vi "Main.vi"() -> ()   [LabVIEW 2020]
uses:
  <vilib>/Instr/_visa.llb/VISA Configure Serial Port (Instr).vi
panel:
  out "Boolean 8":bool=TRUE
  out "Numeric 4":dbl
  out "Numeric 2":dbl
  out "Numeric":dbl
  out "Boolean 7":bool=TRUE
  out "Boolean 6":bool
  out "Boolean 5":bool
  out "Boolean 4":bool
  out "Boolean 3":bool
  out "Boolean 2":bool
  out "Boolean":bool=TRUE
  out "NewVal":bool
  in  "Transmit":bool
  out "Transmitted Data":T1 {"LED" format="%04b"}
  in  "Period":u32
  out "data string":string
  out "Motor Speed":T2(graph)
  out "Waveform Chart":T3(graph)
  out "read buffer":string
  out "Received Data":cluster{i32[], u32}
  in  "Data to transmit":T1 {"LED" format="%04b"}
  out "error out":errorcluster
  in  "VISA resource name":refnum<visa-resource-name>
  in  "Stop":bool
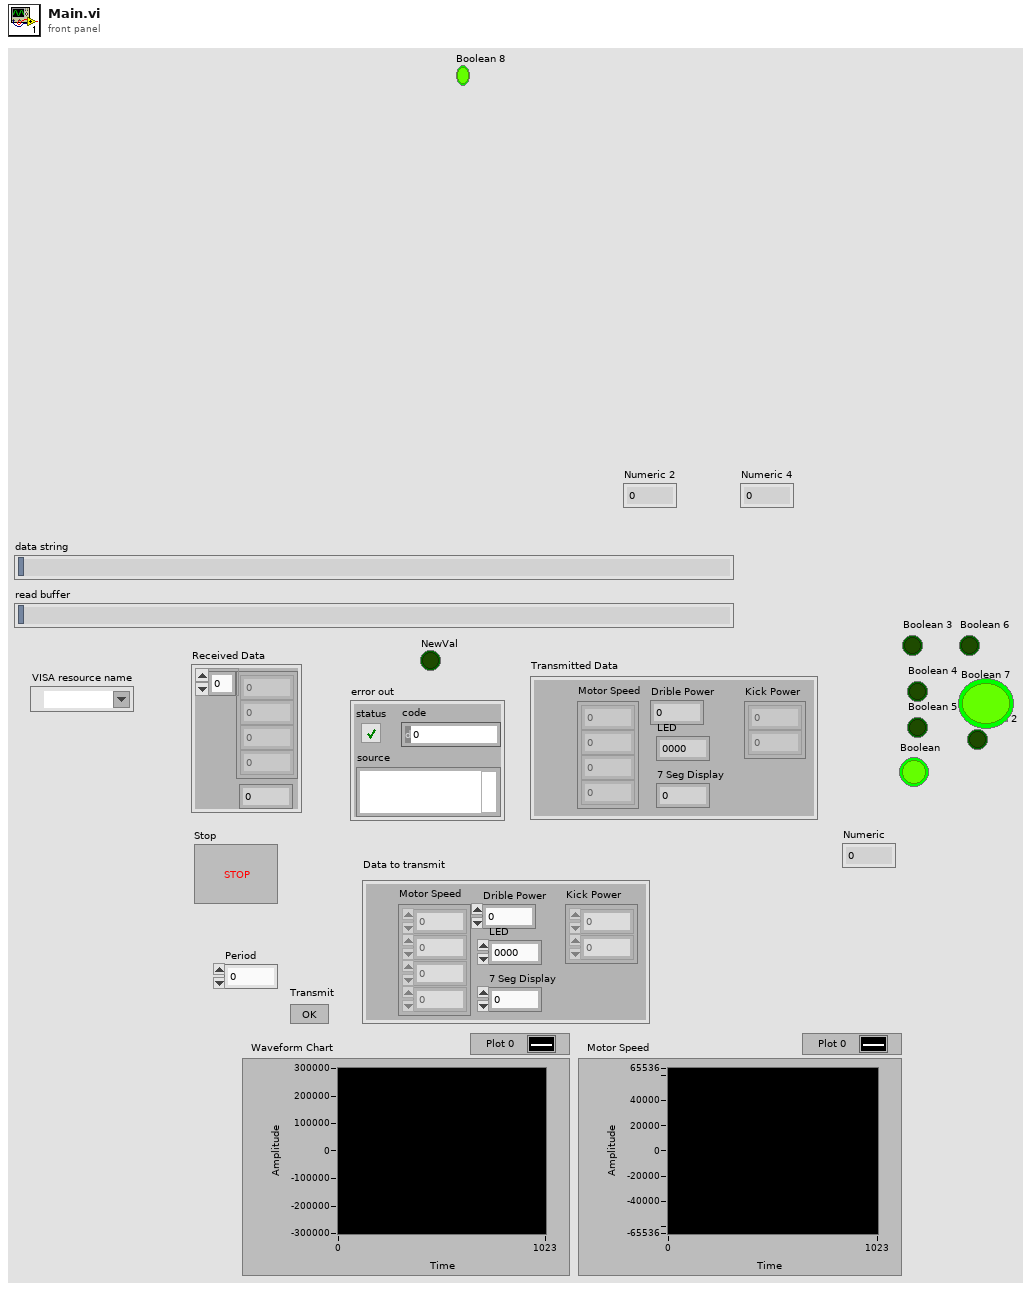
[diagram p1: front panel]
types:
  T1 = cluster{"Motor Speed":i32[], "Drible Power":i32, "LED":u32, "7 Seg Display":u32, "Kick Power":u32[]}
  T2 = cluster{"Motor Speed[0]":i32, "Motor Speed[1]":i32, "Motor Speed[2]":i32, "Motor Speed[3]":i32}
  T3 = cluster{"Encoder[0]":i32, "Encoder[1]":i32, "Encoder[2]":i32, "Encoder[3]":i32}
  T4 = enum16{"big-endian, network order", "native, host order", "little-endian"}
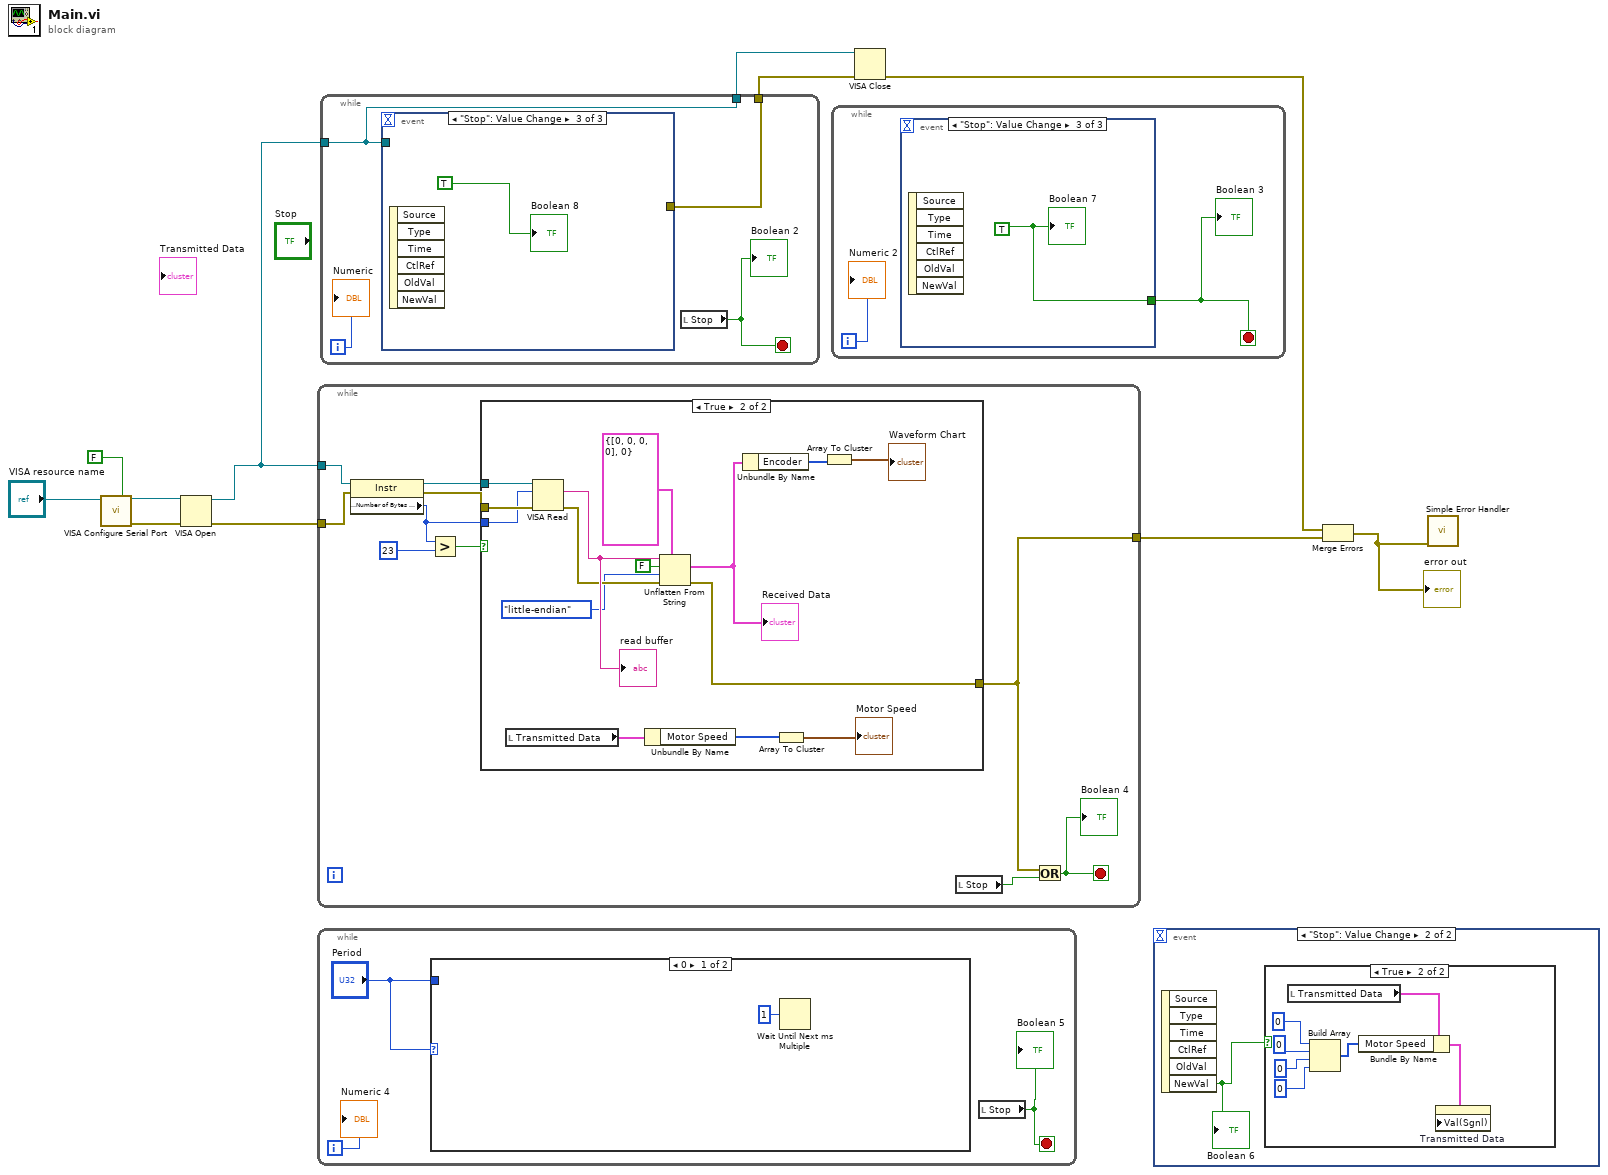
[diagram p0: block diagram]
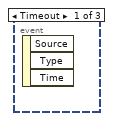
[diagram p2: hidden frame]
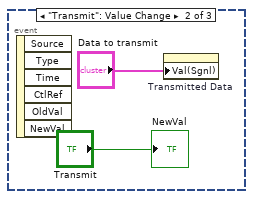
[diagram p3: hidden frame]
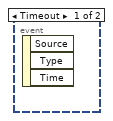
[diagram p4: hidden frame]
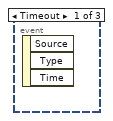
[diagram p6: hidden frame]
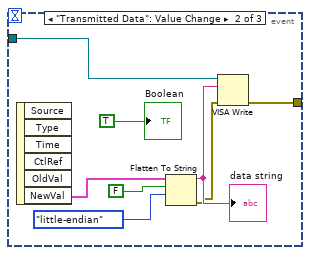
[diagram p7: hidden frame]
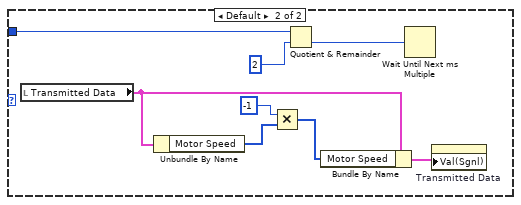
[diagram p9: hidden frame]
diagram:
  n1 = call-poly "VISA Configure Serial Port"("VISA resource name"="VISA resource name", "Enable Termination\nChar (T)"=FALSE ("Enable Termination\nChar (T)")) -> ("VISA resource name out"=w4:refnum<visa-resource-name>, "error out"=w2:errorcluster)  [unwired: 12 in]
  n2 = VISA Open(error in (no error)=w2, VISA resource name=w4) -> (VISA resource name=w10:refnum<visa-resource-name>, error out=w11:errorcluster)  [unwired: 3 in]
  n3 = while {
    tunnel: w10 -> [w17]
    tunnel: w11 -> [w16]
    tunnel: [w13] -> w6
    stop <- w12 stop-if-true
    n4 = property class="Instr"(reference=w17, error in=w16) -> (reference out=w19:refnum<visa-resource-name>, error out=w18:errorcluster, "Serial Settings:Number of Bytes at Serial Port"=w15:u32)
    n5 = Greater?(x=w15, y=u32 23) -> (0:w20:bool)
    n6 = case shown="True" w20 {
      tunnel: w19 -> [_ w37]
      tunnel: w18 -> [w22 w34]
      tunnel: [w22 w32] -> w13
      tunnel: w15 -> [_ w31]
      frame False {
      }
      frame True {
        n7 = local read "Transmitted Data"() -> (w27:T1)
        n8 = VISA Read(VISA resource name=w37, byte count=w31, error in (no error)=w34) -> (read buffer=w36:string, error out=w33:errorcluster)  [unwired: 2 out]
        "read buffer" <- w36
        n9 = Unbundle By Name(w27) -> ("Motor Speed"=w26:i32[])
        n10 = Unflatten From String(type=cluster{"Encoder":i32[], "Button":u32} {"Encoder"=[0, 0, 0, 0], "Button"=0}, binary string=w36, data includes array or string size? (T)=FALSE, byte order (0:big-endian, network order)=T4."little-endian", error in (no error)=w33) -> (value=w28:cluster{"Encoder":i32[], "Button":u32}, error out=w32:errorcluster)  [unwired: 1 out]
        "Received Data" <- w28
        n11 = Unbundle By Name(w28) -> ("Encoder"=w24:i32[])
        n12 = Array To Cluster(array=w26) -> (cluster=→"Motor Speed":T2)
        n13 = Array To Cluster(array=w24) -> (cluster=→"Waveform Chart":T3)
      }
    }
    n14 = local read "Stop"() -> (w14:bool)
    n15 = Or(x=w13, y=w14) -> (x .or. y?=w12:bool)
    "Boolean 4" <- w12
  }
  n16 = while {
    i -> [w38]
    stop <- w39 stop-if-true
    n17 = case shown="0" "Period" {
      tunnel: "Period" -> [_ w47]
      frame 0 {
        n18 = Wait Until Next ms Multiple(millisecond multiple=u32 1) -> ()  [unwired: 1 out]
      }
      frame Default {
        n19 = local read "Transmitted Data"() -> (w45:T1)
        n20 = Unbundle By Name(w45) -> ("Motor Speed"=w44:i32[])
        n21 = Multiply(x=-1, y=w44) -> (x*y=w43:i32[])
        n22 = Quotient & Remainder(x=w47, y=u32 2) -> (floor(x/y)=w48:u32)  [unwired: 1 out]
        n23 = Bundle By Name(cluster=w45, "Motor Speed"=w43) -> (w42:T1)
        n24 = Wait Until Next ms Multiple(millisecond multiple=w48) -> ()  [unwired: 1 out]
        n25 = property on="Transmitted Data" class="Clust (strict)"("Val(Sgnl)"=w42) -> ()  [unwired: 2 in, 2 out]
      }
    }
    n26 = local read "Stop"() -> (w39:bool)
    "Boolean 5" <- w39
    "Numeric 4" <- w38
  }
  n27 = while {
    tunnel: w10 -> [w53]
    tunnel: [w53] -> w9
    tunnel: [w52] -> w8
    i -> [w51]
    stop <- w50 stop-if-true
    n28 = event shown="[2] \"Stop\": Value Change" {
      selector: _ -> [_ _ _]
      dyn-events: _ -> [_ _ _]
      timeout: _ -> [_ _ _]
      tunnel: w53 -> [_ w61 _]
      tunnel: [_ w54 _] -> w52
      event Timeout {
        n29 = event-data() -> ()  [unwired: 1 in, 3 out]
      }
      event "Transmitted Data": Value Change {
        n30 = event-data() -> ("NewVal"=w57:T1)  [unwired: 1 in, 5 out]
        n31 = Flatten To String(anything=w57, prepend array or string size? (T)=FALSE, byte order (0:big-endian, network order)=T4."little-endian") -> (data string=w58:string, error out=w56:errorcluster)  [unwired: 1 in, 1 out]
        "data string" <- w58
        n32 = VISA Write(VISA resource name=w61, write buffer=w58, error in (no error)=w56) -> (error out=w54:errorcluster)  [unwired: 2 out]
        "Boolean" <- TRUE
      }
      event "Stop": Value Change {
        n33 = event-data() -> ()  [unwired: 1 in, 6 out]
        "Boolean 8" <- TRUE
      }
    }
    n34 = local read "Stop"() -> (w50:bool)
    "Boolean 2" <- w50
    "Numeric" <- w51
  }
  n35 = while {
    i -> [w64]
    stop <- w63 stop-if-true
    n36 = event shown="[2] \"Stop\": Value Change" {
      selector: _ -> [_ _ _]
      dyn-events: _ -> [_ _ _]
      timeout: _ -> [_ _ _]
      tunnel: [_ _ w67] -> w63
      event Timeout {
        n37 = event-data() -> ()  [unwired: 1 in, 3 out]
      }
      event "Transmit": Value Change {
        n38 = event-data() -> ()  [unwired: 1 in, 6 out]
        n39 = property on="Transmitted Data" class="Clust (strict)"("Val(Sgnl)"="Data to transmit") -> ()  [unwired: 2 in, 2 out]
        "NewVal" <- "Transmit"
      }
      event "Stop": Value Change {
        w67 = TRUE
        n40 = event-data() -> ()  [unwired: 1 in, 6 out]
        "Boolean 7" <- w67
      }
    }
    "Boolean 3" <- w63
    "Numeric 2" <- w64
  }
  n41 = VISA Close(VISA resource name=w9, error in (no error)=w8) -> (error out=w7:errorcluster)
  n42 = event shown="[1] \"Stop\": Value Change" {
    selector: _ -> [_ _]
    dyn-events: _ -> [_ _]
    timeout: _ -> [_ _]
    event Timeout {
      n43 = event-data() -> ()  [unwired: 1 in, 3 out]
    }
    event "Stop": Value Change {
      n44 = event-data() -> ("NewVal"=w68:bool)  [unwired: 1 in, 5 out]
      "Boolean 6" <- w68
      n45 = case shown="True" w68 {
        frame False {
        }
        frame True {
          n46 = local read "Transmitted Data"() -> (w71:T1)
          n47 = Build Array(0 ("element"), 0 ("element"), 0 ("element"), 0 ("element")) -> (w70:i32[])
          n48 = Bundle By Name(cluster=w71, "Motor Speed"=w70) -> (w69:T1)
          n49 = property on="Transmitted Data" class="Clust (strict)"("Val(Sgnl)"=w69) -> ()  [unwired: 2 in, 2 out]
        }
      }
    }
  }
  n50 = Merge Errors(w7, w6) -> (w5:errorcluster)
  "error out" <- w5
  n51 = call <vilib>:"Simple Error Handler.vi"("error in (no error)"=w5) -> ()  [unwired: 4 in, 5 out]
